vi "New JSON Object (Empty).vi"(8 "error in (no error)":errorcluster) -> (0 "error out":errorcluster, 3 "JSON Value out":refnum<class "JSON Value.lvclass">)   [LabVIEW 2016, in "JSON Value.lvclass"]
doc: "Create a new JSON Object with no specified value."
uses:
  JSON Value.lvclass
  JSON Types.ctl
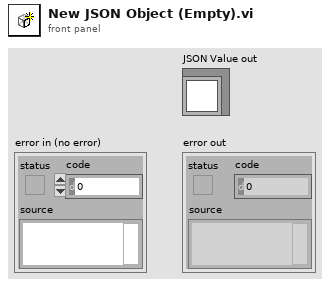
[diagram p1: front panel]
types:
  T1 = typedef "JSON Value.lvclass/JSON Types.ctl" = enum16{"String", "Numeric", "Boolean", "NULL", "Object", "Array"}
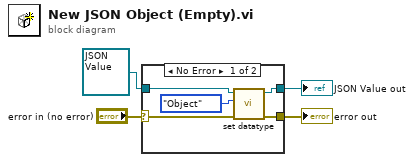
[diagram p0: block diagram]
diagram:
  n1 = case shown="No Error" "error in (no error)" {
    selector: "error in (no error)" -> [w9 w11]
    tunnel: [w8 w11] -> w3
    tunnel: [w6 w10] -> w2
    tunnel: refnum<class "JSON Value.lvclass"> refnum ("JSON Object in") -> [w7 w10]
    frame No Error {
      n2 = call "set datatype.vi"("error in (no error)"=w9, "datatype"=JSON_Types."Object", "JSON Helper in"=w7) -> ("error out"=w8:errorcluster, "JSON Helper out"=w6:refnum<class "JSON Value.lvclass">)  [unwired: 7 in]
    }
    frame Error {
    }
  }
  "error out" <- w3
  "JSON Value out" <- w2
